vi "WPI_PWMERRSetOnUnallocatedChannel.vi"(8 "error in (no error)":errorcluster, 9 "Additional Depth":i32, 10 "PWM Channel":T1) -> (0 "error out":errorcluster)   [LabVIEW 2017]
doc: "This software is licensed. Open the labview\\readme\\WPI Robotics Library Open Source License.txt file for more information."
uses:
  <vilib>/Rock Robotics/SystemInterfaces/DIO/FPGA_DIOPWMChannel.ctl
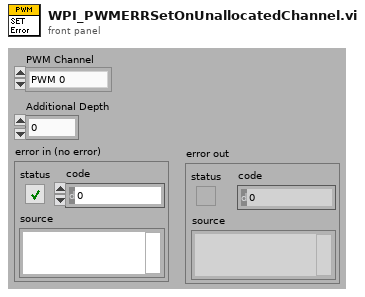
[diagram p1: front panel]
types:
  T1 = typedef "FPGA_DIOPWMChannel.ctl" = enum8{"PWM 0", "PWM 1", "PWM 2", "PWM 3", "PWM 4", "PWM 5", "PWM 6", "PWM 7", "PWM 8", "PWM 9", "PWM MXP 0", "PWM MXP 1", "PWM MXP 2", "PWM MXP 3", "PWM MXP 4", "PWM MXP 5", "PWM MXP 6", "PWM MXP 7", "PWM MXP 8", "PWM MXP 9", "Invalid"}
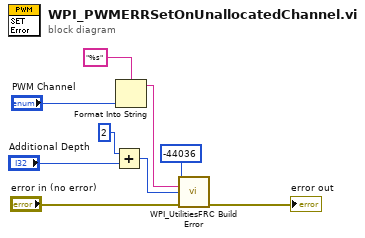
[diagram p0: block diagram]
diagram:
  n1 = Add(x=2 ("chain levels to remove (1)"), y="Additional Depth") -> (x+y=w5:i32)
  n2 = Format Into String(format string="%s", "PWM Channel") -> (resulting string=w1:string)  [unwired: 2 in, 1 out]
  n3 = call <vilib>:"WPI_UtilitiesFRC Build Error.vi"("error code"=-44036 ("code"), "extra error text"=w1, "chain levels to remove (1)"=w5, "error in (no error)"="error in (no error)") -> ("error out"=→"error out":errorcluster)  [unwired: 1 in, 10 out]
